vi "Stand Alone Temp.vi"() -> ()   [LabVIEW 2017, in "Temperature Controller.lvclass"]
uses:
  Temperature Controller.lvclass
  Utility Classes/Instrument/Instrument.lvclass
  Global/Relative Sound Files.vi
  HV Slide Indicator.ctl
panel:
  in  "Instrument in":refnum<class "Instrument.lvclass">
  in  "Temperature Controller.lvclass":refnum<class "Temperature Controller.lvclass">
  in  "warnON":bool caption="Warn On"
  in  "greater":bool caption="Temp Greater?"
  in  "warn":dbl caption="Warn at"
  out "nv%":dbl(slide) caption="NV" scale=0.0..100.0
  out "heater%":dbl(slide) caption="Heater" scale=0.0..100.0
  out "active":bool
  out "ok":bool
  in  "exit":bool
  out "temp":dbl
  # "On"
  # "K"
  # "K"
  # "Status"
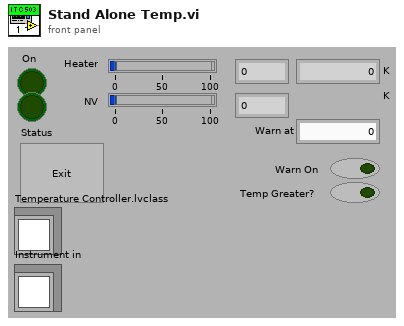
[diagram p1: front panel]
types:
  T1 = typedef "Temperature Controller.lvclass/HV Slide Indicator.ctl" = dbl
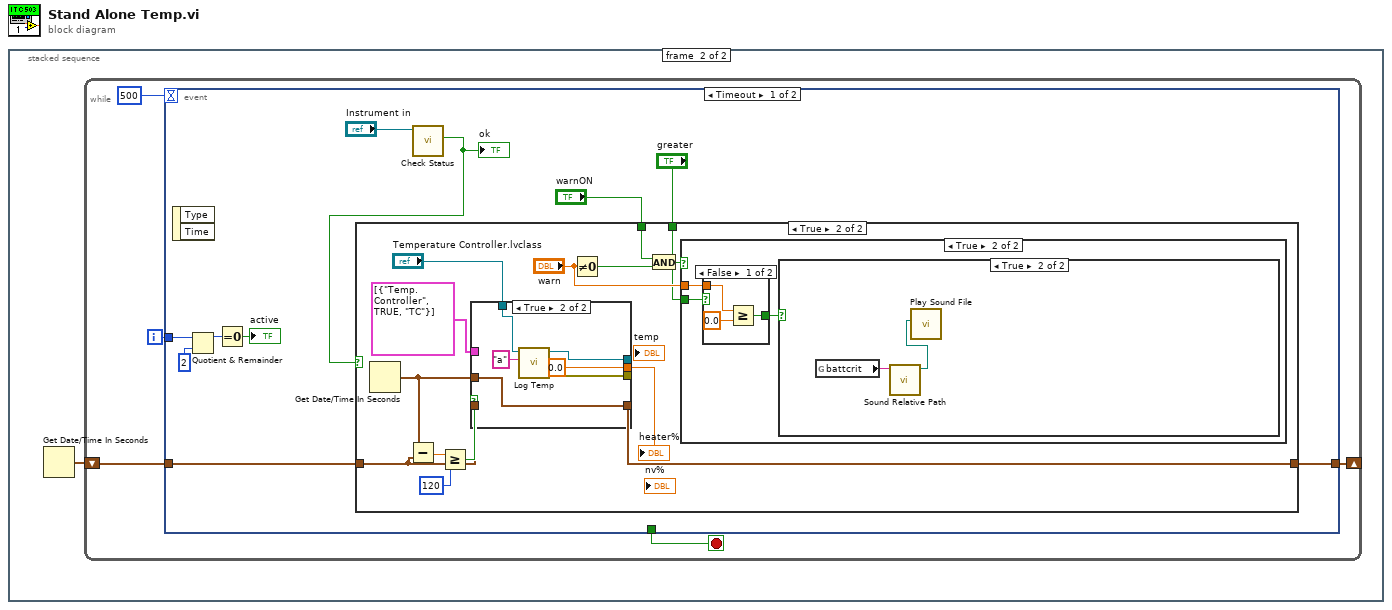
[diagram p0: block diagram]
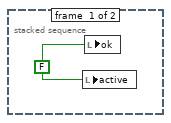
[diagram p2: hidden frame]
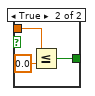
[diagram p5: hidden frame]
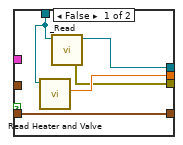
[diagram p7: hidden frame]
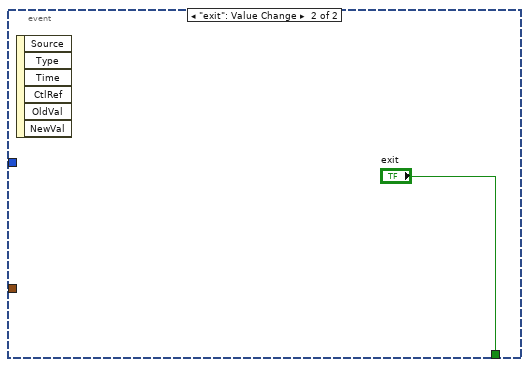
[diagram p8: hidden frame]
diagram:
  n1 = stacked-sequence {
    frame #0 {
      w1 = FALSE
      n2 = local write "active"(w1) -> ()
      n3 = local write "ok"(w1) -> ()
    }
    frame #1 {
      n4 = Get Date/Time In Seconds() -> (seconds since 1Jan1904=w2:timestamp)
      n5 = while {
        shift-right: [w3] -> _
        shift-left: w2 -> [w4]
        i -> [w5]
        stop <- w7 stop-if-true
        n6 = event shown="[0] Timeout" {
          selector: _ -> [_ _]
          dyn-events: _ -> [_ _]
          timeout: 500 -> [_ _]
          tunnel: [_ "exit"] -> w7
          tunnel: w5 -> [w17 _]
          tunnel: w4 -> [w13 _]
          tunnel: [w12 _] -> w3
          event Timeout {
            n7 = event-data() -> ()  [unwired: 3 out]
            n8 = Quotient & Remainder(x=w17, y=2) -> (x-y*floor(x/y)=w15:i32)  [unwired: 1 out]
            n9 = Equal To 0?(x=w15) -> (x = 0?=→"active":bool)
            n10 = call-dynamic "Check Status.vi"("Instrument in"="Instrument in") -> ("Ready?"=w9:bool)  [unwired: 7 in, 3 out]
            "ok" <- w9
            n11 = case shown="True" w9 {
              tunnel: w13 -> [w18 w27]
              tunnel: [w18 w26] -> w12
              tunnel: "greater" -> [_ w23]
              tunnel: "warnON" -> [_ w20]
              frame False {
              }
              frame True {
                n12 = Get Date/Time In Seconds() -> (seconds since 1Jan1904=w28:timestamp)
                n13 = Subtract(x=w28, y=w27) -> (x-y=w32:dbl)
                n14 = Greater Or Equal?(x=w32, y=120) -> (x >= y?=w30:bool)
                n15 = case shown="True" w30 {
                  tunnel: [w48 w52] -> _
                  tunnel: cluster{string, bool, string}[] [{"Temp. Controller", TRUE, "TC"}] -> [_ _]
                  tunnel: w28 -> [_ w54]
                  tunnel: w27 -> [w47 _]
                  tunnel: [w47 w54] -> w26
                  tunnel: [w46 T1 0.0 ("heater%")] -> w25
                  tunnel: [w45 w53] -> _
                  tunnel: "Temperature Controller.lvclass" -> [w44 w49]
                  frame False {
                    n16 = call-dynamic "Read Heater and Valve.vi"("Temperature Controller in"=w44) -> ("heater%"=w46:T1)  [unwired: 7 in, 3 out]
                    n17 = call-dynamic "_Read.vi"("Temperature Controller.lvclass"=w44) -> ("error out"=w45:errorcluster, "Temperature Controller out"=w48:refnum<class "Temperature Controller.lvclass">)  [unwired: 8 in, 1 out]
                  }
                  frame True {
                    n18 = call-dynamic "Log Temp.vi"("Status string"="a", "Temperature Controller in"=w49) -> ("error out"=w53:errorcluster, "Temperature Controller out"=w52:refnum<class "Temperature Controller.lvclass">)  [unwired: 8 in]
                  }
                }
                "heater%" <- w25
                n19 = Not Equal To 0?(x="warn") -> (x != 0?=w21:bool)
                n20 = And(x=w20, y=w21) -> (x .and. y?=w22:bool)
                n21 = case shown="True" w22 {
                  tunnel: "warn" -> [_ w35]
                  tunnel: w23 -> [_ w33]
                  frame False {
                  }
                  frame True {
                    n22 = case shown="False" w33 {
                      tunnel: w35 -> [w37 w41]
                      tunnel: [w38 w40] -> w34
                      frame False {
                        n23 = Greater Or Equal?(x=w37, y=0.0) -> (x >= y?=w38:bool)
                      }
                      frame True {
                        n24 = Less Or Equal?(x=w41, y=0.0) -> (x <= y?=w40:bool)
                      }
                    }
                    n25 = case shown="True" w34 {
                      frame False {
                      }
                      frame True {
                        n26 = global read "Relative Sound Files.vi" "battcrit"() -> (w43:string)
                        n27 = call "Sound Relative Path.vi"("Sound"=w43) -> ("Relative Path"=w42:path)  [unwired: 10 in]
                        n28 = call <vilib>:"Play Sound File.vi"("path"=w42) -> ()  [unwired: 3 in, 8 out]
                      }
                    }
                  }
                }
              }
            }
          }
          event "exit": Value Change {
            n29 = event-data() -> ()  [unwired: 7 out]
          }
        }
      }
    }
  }
